vi "Sinus_Build_subVI.vi"(6 "Amplitude":dbl=1.0 format="%0.2p", 7 "Desired Frequency":dbl format="%#_13g", 8 "error in":errorcluster, 9 "Cycles per Buffer":i32, 10 "Samples per Buffer":i32, 11 "task in":refnum<k21>) -> (0 "error out":errorcluster, 2 "Waveform":waveform(dbl), 3 "task out":refnum<k21>)   [LabVIEW 2020]
doc: "This VI builds sinus waveform for DAQ generating (Analog Output). It also configures DAQmx Timing."
uses:
  <resource>/objmgr/daqmx.rc
  <vilib>/measure/NI_MABase.lvlib
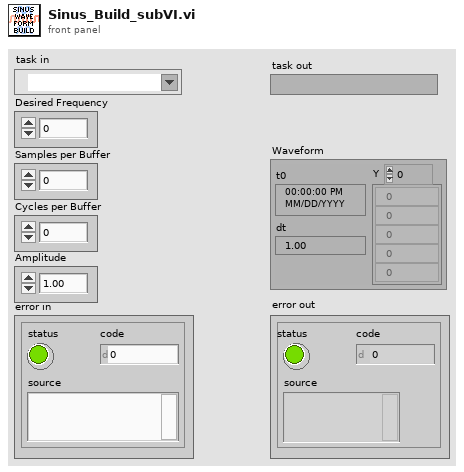
[diagram p1: front panel]
types:
  T1 = enum16{"Sine Wave", "Triangle Wave", "Square Wave", "Sawtooth Wave"}
  T2 = cluster{"SampClk.Rate":dbl, "Samples per Buffer":i32}
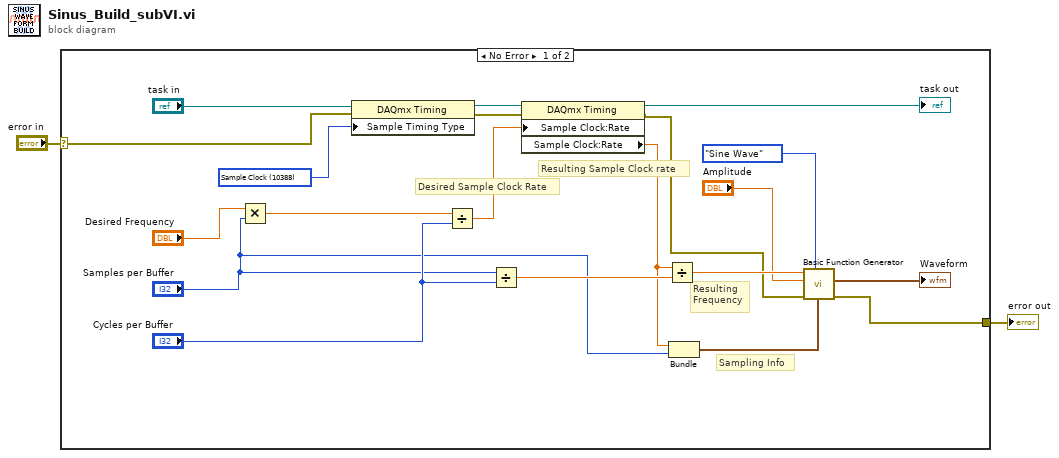
[diagram p0: block diagram]
diagram:
  n1 = case shown="No Error" "error in" {
    selector: "error in" -> [w3 w23]
    tunnel: [w4 w23] -> w2
    frame No Error {
      w21 = 10388 items=["Sample Clock"=10388, "Burst Handshake"=12548, "Handshake"=10389, "Implicit"=10451, "On Demand"=10390, "Change Detection"=12504, "Pipelined Sample Clock"=14668] ("SampTimingType")
      # "Sampling Info"
      # "Resulting\nFrequency"
      # "Resulting Sample Clock rate"
      # "Desired Sample Clock Rate"
      n2 = Multiply(x="Desired Frequency", y="Samples per Buffer") -> (x*y=w16:dbl)
      n3 = property class="DAQmx Timing"(reference="task in", error in=w3, "Sample Timing Type"=w21) -> (reference out=w20:refnum<k21>, error out=w19:errorcluster)
      n4 = Divide(x=w16, y="Cycles per Buffer") -> (x/y=w15:dbl)
      n5 = Divide(x="Samples per Buffer", y="Cycles per Buffer") -> (x/y=w12:dbl)
      n6 = property class="DAQmx Timing"(reference=w20, error in=w19, "Sample Clock:Rate"=w15) -> (reference out=→"task out":refnum<k21>, error out=w9:errorcluster, "Sample Clock:Rate"=w8:dbl)
      n7 = Divide(x=w8, y=w12) -> (x/y=w11:dbl)
      n8 = Bundle("SampClk.Rate"=w8, "Samples per Buffer"="Samples per Buffer") -> (w6:T2)  [unwired: 1 in]
      n9 = call <vilib>:"Basic Function Generator.vi"("sampling info"=w6, "signal type"=T1."Sine Wave", "error in (no error)"=w9, "amplitude"="Amplitude", "frequency"=w11) -> ("error out"=w4:errorcluster, "signal out"=→"Waveform":waveform(dbl))  [unwired: 4 in, 1 out]
    }
    frame Error {
    }
  }
  "error out" <- w2
